vi "recreateTree.vi"(0 "Tree ref":refnum<vi>, 1 "Rig path":string, 2 "Calibration path":string, 3 "Stimulus path":string, 5 "parent tag":string, 7 "Active Item:Indent Level":i32, 9 "new tag":string, 11 "Symbol":i32=20, 12 "Req":string, 13 "Element Name":string, 14 "Analysis script path":string) -> ()   [LabVIEW 2010]
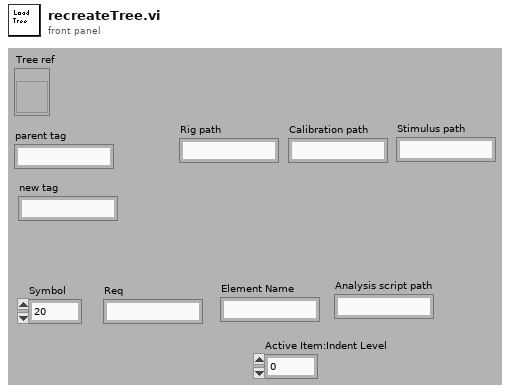
[diagram p1: front panel]
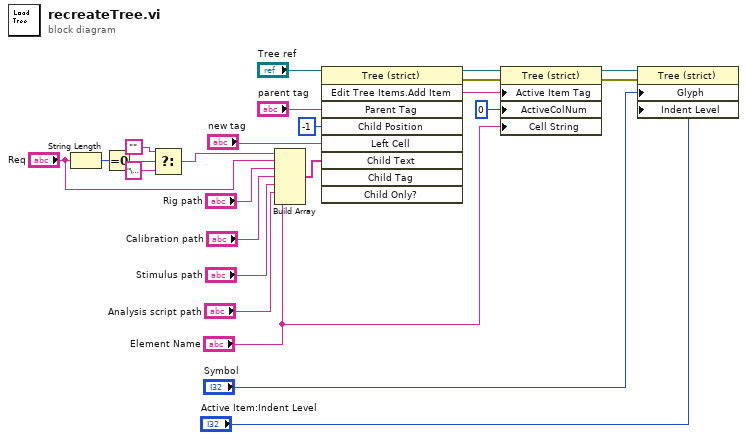
[diagram p0: block diagram]
diagram:
  n1 = String Length(string="Req") -> (length=w6:i32)
  n2 = Equal To 0?(x=w6) -> (x = 0?=w5:bool)
  n3 = Select(t="", s=w5, f="\u0007") -> (s? t:f=w2:string)
  n4 = Build Array(w2, "Req", "Rig path", "Calibration path", "Stimulus path", "Analysis script path", "Element Name") -> (w17:string[])
  n5 = invoke on="Invoke Node" class="Tree (strict)" method="Edit Tree Items.Add Item"(reference="Tree ref", "Parent Tag"="parent tag", "Child Position"=-1, "Left Cell"="new tag", "Child Text"=w17) -> (reference out=w23:refnum<vi>, error out=w21:errorcluster, "Edit Tree Items:Add Item"=w20:string)  [unwired: 4 in, 6 out]
  n6 = property on="Property Node" class="Tree (strict)"(reference=w23, error in=w21, "Active Item Tag"=w20, "ActiveColNum"=0 ("Active Item:Row Number"), "Cell String"="Element Name") -> (reference out=w10:refnum<vi>, error out=w9:errorcluster)
  n7 = property on="Property Node" class="Tree (strict)"(reference=w10, error in=w9, "Glyph"="Symbol", "Indent Level"="Active Item:Indent Level") -> ()  [unwired: 2 out]
